vi "Rohde & Schwarz VNA Read External Trigger Mode.vi"(6 "Channel":i8=1 min=1 max=99 step=1, 7 "Rohde & Schwarz VNA":T1, 8 "error in (no error)":errorcluster, 11 "VISA Resource Name":refnum<visa-resource-name>) -> (0 "error out":errorcluster, 2 "Ext. Trigger Mode":T2, 3 "dup VISA Resource Name":refnum<visa-resource-name>)   [LabVIEW 2011]
doc: "This VI for the HP8753B Network Analyzers reads the stimulus values. Except when performing log sweeps and freq list sweeps, this VI uses the start and stop values and the number of points to calcuate the stimulus values."
uses:
  TypeDefs/Rohde & Schwarz VNA External Trigger Mode.ctl
  TypeDefs/Rohde & Schwarz VNA Instrument Info.ctl
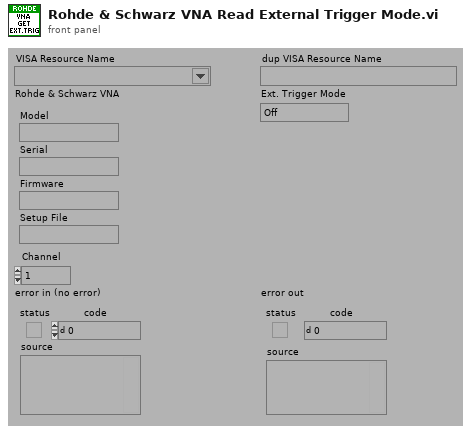
[diagram p1: front panel]
types:
  T1 = typedef "Rohde & Schwarz VNA Instrument Info.ctl" = cluster{"Model":string, "Serial":string, "Firmware":string, "Setup File":string}
  T2 = typedef "Rohde & Schwarz VNA External Trigger Mode.ctl" = enum16{"Off", "Rising Edge", "Falling Edge", "Periodic", "Manual"}
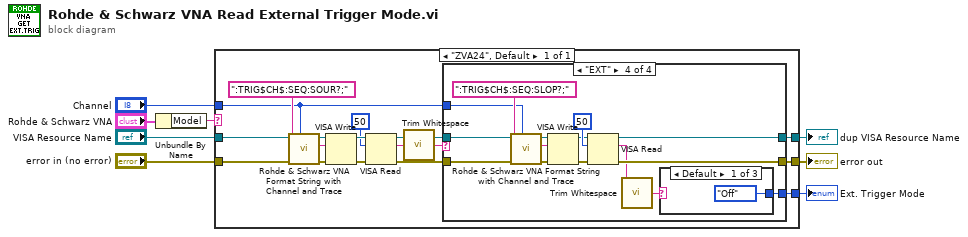
[diagram p0: block diagram]
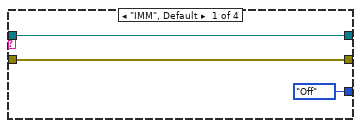
[diagram p2: hidden frame]
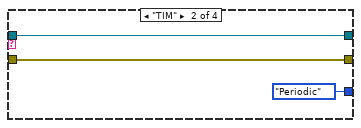
[diagram p3: hidden frame]
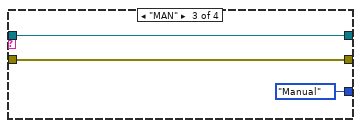
[diagram p4: hidden frame]
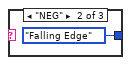
[diagram p5: hidden frame]
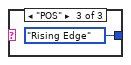
[diagram p6: hidden frame]
diagram:
  n1 = Unbundle By Name("Rohde & Schwarz VNA") -> ("Model"=w3:string)
  n2 = case shown="\"ZVA24\", Default" w3 {
    tunnel: "error in (no error)" -> [w19]
    tunnel: [w11] -> w7
    tunnel: "VISA Resource Name" -> [w20]
    tunnel: [w12] -> w5
    tunnel: "Channel" -> [w9]
    tunnel: [w10] -> w1
    frame "ZVA24", Default {
      n3 = call "Rohde & Schwarz VNA Format String with Channel and Trace.vi"("Channel"=w9, "String"=":TRIG$CH$:SEQ:SOUR?;") -> ("String Out"=w15:string)  [unwired: 1 in, 6 out]
      n4 = VISA Write(VISA resource name=w20, write buffer=w15, error in (no error)=w19) -> (VISA resource name out=w23:refnum<visa-resource-name>, error out=w22:errorcluster)  [unwired: 1 out]
      n5 = VISA Read(VISA resource name=w23, byte count=u32 50, error in (no error)=w22) -> (VISA resource name out=w13:refnum<visa-resource-name>, read buffer=w18:string, error out=w14:errorcluster)  [unwired: 1 out]
      n6 = call <vilib>:"Trim Whitespace.vi"("string"=w18) -> ("trimmed string"=w17:string)  [unwired: 1 in]
      n7 = case shown="\"EXT\"" w17 {
        tunnel: w14 -> [w26 w29 w32 w40]
        tunnel: w13 -> [w25 w28 w31 w41]
        tunnel: [w25 w28 w31 w38] -> w12
        tunnel: [w26 w29 w32 w39] -> w11
        tunnel: [Rohde_&_Schwarz_VNA_External_Trigger_Mode."Off" ("Ext. Trigger Mode") Rohde_&_Schwarz_VNA_External_Trigger_Mode."Periodic" ("Ext. Trigger Mode") Rohde_&_Schwarz_VNA_External_Trigger_Mode."Manual" ("Ext. Trigger Mode") w33] -> w10
        tunnel: w9 -> [_ _ _ w36]
        frame "IMM", Default {
        }
        frame "TIM" {
        }
        frame "MAN" {
        }
        frame "EXT" {
          n8 = call "Rohde & Schwarz VNA Format String with Channel and Trace.vi"("Channel"=w36, "String"=":TRIG$CH$:SEQ:SLOP?;") -> ("String Out"=w45:string)  [unwired: 1 in, 6 out]
          n9 = VISA Write(VISA resource name=w41, write buffer=w45, error in (no error)=w40) -> (VISA resource name out=w42:refnum<visa-resource-name>, error out=w43:errorcluster)  [unwired: 1 out]
          n10 = VISA Read(VISA resource name=w42, byte count=u32 50, error in (no error)=w43) -> (VISA resource name out=w38:refnum<visa-resource-name>, read buffer=w35:string, error out=w39:errorcluster)  [unwired: 1 out]
          n11 = call <vilib>:"Trim Whitespace.vi"("string"=w35) -> ("trimmed string"=w34:string)  [unwired: 1 in]
          n12 = case shown="Default" w34 {
            tunnel: [Rohde_&_Schwarz_VNA_External_Trigger_Mode."Off" ("Ext. Trigger Mode") Rohde_&_Schwarz_VNA_External_Trigger_Mode."Falling Edge" ("Ext. Trigger Mode") Rohde_&_Schwarz_VNA_External_Trigger_Mode."Rising Edge" ("Ext. Trigger Mode")] -> w33
            frame Default {
            }
            frame "NEG" {
            }
            frame "POS" {
            }
          }
        }
      }
    }
  }
  "dup VISA Resource Name" <- w5
  "error out" <- w7
  "Ext. Trigger Mode" <- w1
